vi "MUSIQC_trap_control.vi"() -> ()   [LabVIEW 2009]
uses:
  <vilib>/DAQmx/configure/timing.llb/DAQmx Timing (Implicit).vi
  <vilib>/DAQmx/create/channels.llb/DAQmx Create Channel (CO-Pulse Generation-Frequency).vi
  <vilib>/DAQmx/configure/timing.llb/DAQmx Timing (Sample Clock).vi
  <vilib>/DAQmx/create/channels.llb/DAQmx Create Channel (CI-Count Edges).vi
  <vilib>/DAQmx/read.llb/DAQmx Read (Counter U32 1Chan 1Samp).vi
  <vilib>/Utility/file.llb/Write To Spreadsheet File (I64).vi
  Program Files/National Instruments/LabVIEW 2009/resource/objmgr/daqmx.rc
  <vilib>/Analysis/NI_AALBase.lvlib
panel:
  out "Change with UV":i32(graph)
  in  "snap":bool
  in  "Threshold":u32
  in  "Auto Load":bool
  in  "Oven":bool
  in  "UV":bool=TRUE
  in  "UV Interval (s)":dbl
  in  "RF":bool
  in  "Blue":bool
  in  "Red":bool
  out "Mean/Variance":dbl
  out "Variance":dbl format="%0.2f"
  out "Mean":dbl format="%0.2f"
  in  "Samples per block":i32=100 min=1 step=1
  in  "Sample Time":dbl=0.02 step=0.0001
  in  "stop":bool
  out "PMT Counts":cluster{"mean":dbl, u32, i32}(graph)
  out "Counts total":dbl
  # "Trap 1"
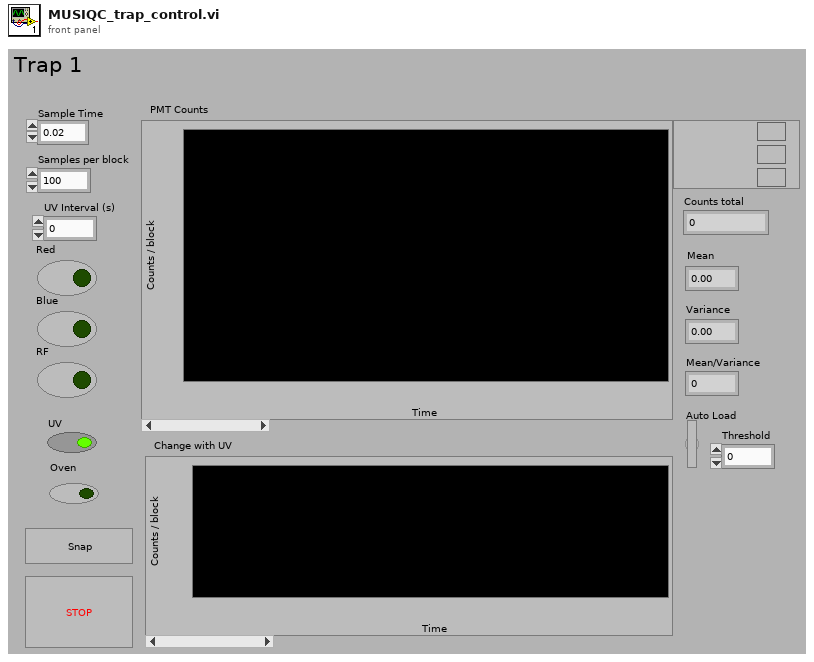
[diagram p1: front panel]
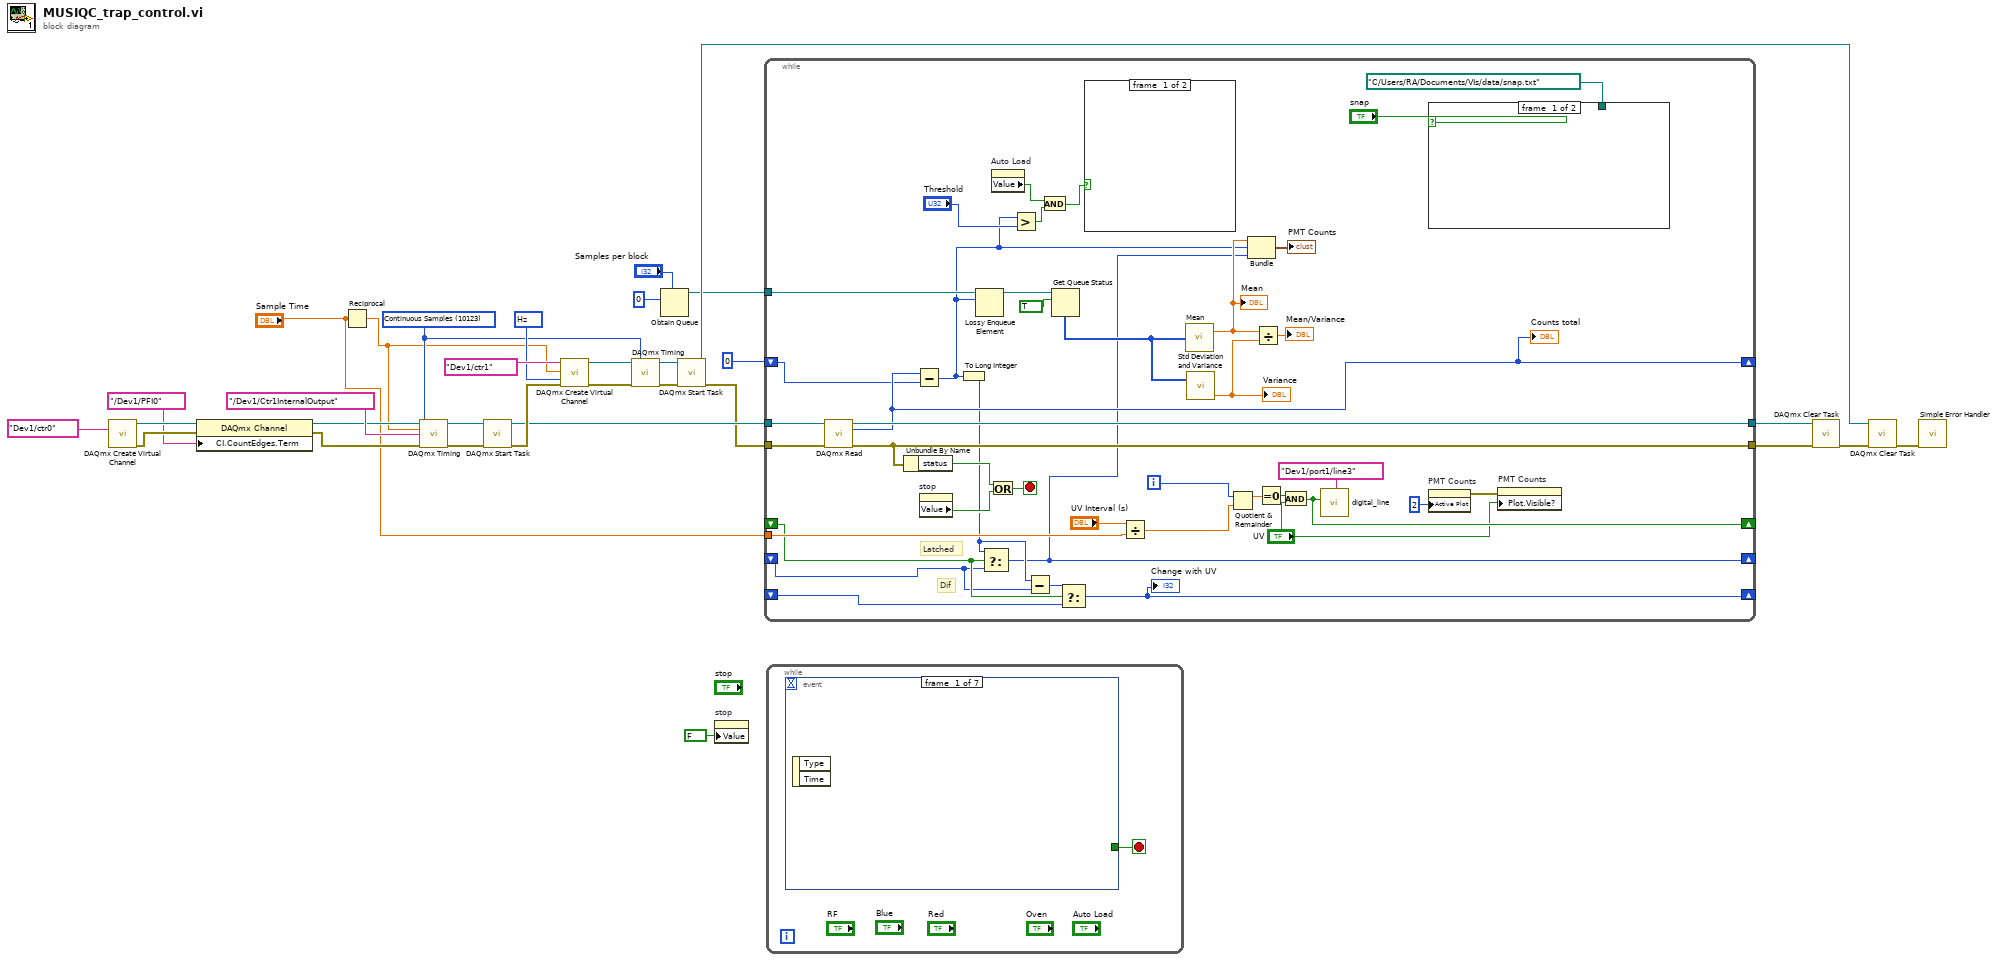
[diagram p0: block diagram]
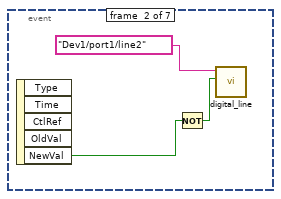
[diagram p2: hidden frame]
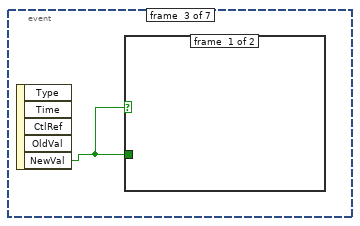
[diagram p3: hidden frame]
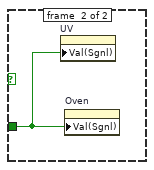
[diagram p4: hidden frame]
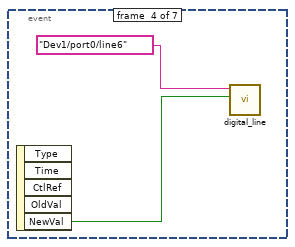
[diagram p5: hidden frame]
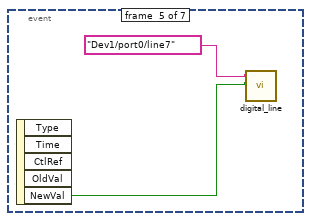
[diagram p6: hidden frame]
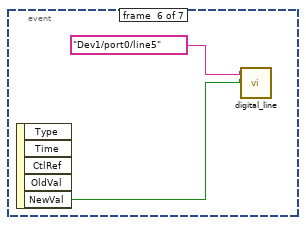
[diagram p7: hidden frame]
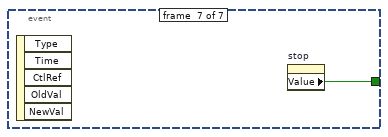
[diagram p8: hidden frame]
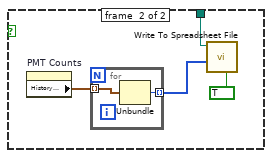
[diagram p9: hidden frame]
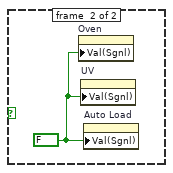
[diagram p10: hidden frame]
diagram:
  w27 = 10373 items=["Hz"=10373] ("units")
  w3 = 10123 items=["Finite Samples"=10178, "Continuous Samples"=10123, "Hardware Timed Single Point"=12522] ("sample mode")
  n1 = call-poly <vilib>:"DAQmx Create Virtual Channel.vi"("counter"=tag "Dev1/ctr0") -> ("task out"=w12:refnum<k21>, "error out"=w11:errorcluster)  [unwired: 13 in]
  n2 = property class="DAQmx Channel"(reference=w12, error in=w11, "CI.CountEdges.Term"=tag "/Dev1/PFI0") -> (reference out=w14:refnum<k21>, error out=w13:errorcluster)
  n3 = Reciprocal(x="Sample Time") -> (1/x=w2:dbl)
  n4 = call-poly <vilib>:"DAQmx Timing.vi"("task/channels in"=w14, "sample mode"=w3, "rate"=w2, "source"=tag "/Dev1/Ctr1InternalOutput", "error in"=w13) -> ("task out"=w30:refnum<k21>, "error out"=w29:errorcluster)  [unwired: 9 in]
  n5 = call <vilib>:"DAQmx Start Task.vi"("task/channels in"=w30, "error in"=w29) -> ("task out"=w17:refnum<k21>, "error out"=w21:errorcluster)  [unwired: 12 in]
  n6 = call-poly <vilib>:"DAQmx Create Virtual Channel.vi"("frequency"=w2, "counter"=tag "Dev1/ctr1", "units"=w27, "error in"=w21) -> ("task out"=w25:refnum<k21>, "error out"=w24:errorcluster)  [unwired: 10 in]
  n7 = call-poly <vilib>:"DAQmx Timing.vi"("task/channels in"=w25, "sample mode"=w3, "error in"=w24) -> ("task out"=w23:refnum<k21>, "error out"=w22:errorcluster)  [unwired: 11 in]
  n8 = Obtain Queue(max queue size (-1, unlimited)="Samples per block", element data type=u32 0) -> (queue out=w7:refnum<queue>)  [unwired: 3 in, 2 out]
  n9 = call <vilib>:"DAQmx Start Task.vi"("task/channels in"=w23, "error in"=w22) -> ("task out"=w16:refnum<k21>, "error out"=w15:errorcluster)  [unwired: 12 in]
  n10 = property on="stop" class="Bool (strict)"("Value"=FALSE ("stop")) -> ()  [unwired: 2 in, 2 out]
  n11 = while {
    shift-right: [w44] -> _
    shift-left: u32 0 -> [w43]
    tunnel: [w71] -> w19
    tunnel: [w70] -> w18
    tunnel: w17 -> [w69]
    tunnel: w15 -> [w68]
    tunnel: w7 -> [w67]
    tunnel: "Sample Time" -> [w48]
    shift-right: [w45] -> _
    shift-left: _ -> [w42]
    shift-right: [w34] -> _
    shift-left: _ -> [w41]
    shift-right: [w39] -> _
    shift-left: _ -> [w37]
    i -> [w49]
    stop <- w73 stop-if-true
    # "Dif"
    # "Latched"
    n12 = call-poly <vilib>:"DAQmx Read.vi"("task/channels in"=w69, "error in"=w68) -> ("task out"=w70:refnum<k21>, "data"=w44:u32, "error out"=w71:errorcluster)  [unwired: 11 in]
    "Counts total" <- w44
    n13 = Unbundle By Name(w71) -> ("status"=w72:bool)
    n14 = Subtract(x=w44, y=w43) -> (x-y=w35:u32)
    n15 = property on="stop" class="Bool (strict)"() -> ("Value"=w60:bool)  [unwired: 2 in, 2 out]
    n16 = To Long Integer(number=w35) -> (32bit integer=w38:i32)
    n17 = Lossy Enqueue Element(queue=w67, element=w35) -> (queue out=w66:refnum<queue>)  [unwired: 1 in, 3 out]
    n18 = Select(t=w38, s=w42, f=w41) -> (s? t:f=w34:i32)
    n19 = Or(x=w72, y=w60) -> (x .or. y?=w73:bool)
    n20 = property on="Auto Load" class="Bool (strict)"() -> ("Value"=w57:bool)  [unwired: 2 in, 2 out]
    n21 = Greater?(x=w35, y="Threshold") -> (0:w58:bool)
    n22 = Subtract(x=w38, y=w41) -> (x-y=w40:i32)
    n23 = And(x=w57, y=w58) -> (x .and. y?=w56:bool)
    n24 = Get Queue Status(queue=w66, return elements? (F)=TRUE) -> (elements=w54:u32[])  [unwired: 1 in, 7 out]
    n25 = Select(t=w40, s=w42, f=w37) -> (s? t:f=w39:i32)
    "Change with UV" <- w39
    n26 = case shown="True" w56 {
      frame #0 {
      }
      frame #1 {
        w80 = FALSE ("Auto Load")
        n27 = property on="Oven" class="Bool (strict)"("Val(Sgnl)"=w80) -> ()  [unwired: 2 in, 2 out]
        n28 = property on="UV" class="Bool (strict)"("Val(Sgnl)"=w80) -> ()  [unwired: 2 in, 2 out]
        n29 = property on="Auto Load" class="Bool (strict)"("Val(Sgnl)"=w80) -> ()  [unwired: 2 in, 2 out]
      }
    }
    n30 = Divide(x="UV Interval (s)", y=w48) -> (x/y=w47:dbl)
    n31 = call <vilib>:"Mean.vi"("X"=w54) -> ("mean"=w61:dbl)  [unwired: 1 out]
    "Mean" <- w61
    n32 = call <vilib>:"Std Deviation and Variance.vi"("X"=w54) -> ("variance"=w64:dbl)  [unwired: 1 in, 2 out]
    "Variance" <- w64
    n33 = Quotient & Remainder(x=w49, y=w47) -> (x-y*floor(x/y)=w52:dbl)  [unwired: 1 out]
    n34 = Bundle("mean"=w61, w35, w34) -> (→"PMT Counts":cluster{"mean":dbl, u32, i32})  [unwired: 1 in]
    n35 = Divide(x=w61, y=w64) -> (x/y=→"Mean/Variance":dbl)
    n36 = Equal To 0?(x=w52) -> (x = 0?=w50:bool)
    n37 = And(x=w50, y="UV") -> (x .and. y?=w45:bool)
    n38 = call "digital_line.vi"("NewVal"=w45, "lines"=tag "Dev1/port1/line3") -> ()  [unwired: 2 in]
    n39 = property on="PMT Counts" class="WFChart (strict)"("Active Plot"=u32 2) -> (error out=w32:errorcluster)  [unwired: 2 in, 1 out]
    n40 = case shown="True" "snap" {
      tunnel: path "C:/Users/RA/Documents/VIs/data/snap.txt" ("file path (dialog if empty)") -> [_ w76]
      frame #0 {
      }
      frame #1 {
        n41 = property on="PMT Counts" class="WFChart (strict)"() -> ("History Data"=w75:cluster{"mean":dbl, u32, i32}[])  [unwired: 2 in, 2 out]
        n42 = for {
          tunnel: w75 -> [w79] mode=indexing
          tunnel: [w78] -> w74 mode=indexing
          n43 = Unbundle(w79) -> (w78:u32)  [unwired: 2 out]
        }
        n44 = call-poly <vilib>:"Write To Spreadsheet File.vi"("transpose? (no:F)"=TRUE, "1D data"=w74, "file path (dialog if empty)"=w76) -> ()  [unwired: 5 in, 1 out]
      }
    }
    n45 = property on="PMT Counts" class="WFChart (strict)"(error in=w32, "Plot.Visible?"="UV") -> ()  [unwired: 1 in, 2 out]
  }
  n46 = while {
    stop <- w81 stop-if-true
    n47 = event shown="[3] \"Red\": Value Change" {
      selector: _ -> [_ _ _ _ _ _ _]
      dyn-events: _ -> [_ _ _ _ _ _ _]
      timeout: _ -> [_ _ _ _ _ _ _]
      tunnel: [_ _ _ _ _ _ w93] -> w81
      event #0 {
        n48 = event-data() -> ()  [unwired: 1 in, 2 out]
      }
      event #1 {
        n49 = event-data() -> ("NewVal"=w83:bool)  [unwired: 1 in, 4 out]
        n50 = Not(x=w83) -> (.not. x?=w82:bool)
        n51 = call "digital_line.vi"("NewVal"=w82, "lines"=tag "Dev1/port1/line2") -> ()  [unwired: 2 in]
      }
      event #2 {
        n52 = event-data() -> ("NewVal"=w85:bool)  [unwired: 1 in, 4 out]
        n53 = case shown="True" w85 {
          tunnel: w85 -> [_ w86]
          frame #0 {
          }
          frame #1 {
            n54 = property on="UV" class="Bool (strict)"("Val(Sgnl)"=w86) -> ()  [unwired: 2 in, 2 out]
            n55 = property on="Oven" class="Bool (strict)"("Val(Sgnl)"=w86) -> ()  [unwired: 2 in, 2 out]
          }
        }
      }
      event #3 {
        n56 = event-data() -> ("NewVal"=w87:bool)  [unwired: 1 in, 4 out]
        n57 = call "digital_line.vi"("NewVal"=w87, "lines"=tag "Dev1/port0/line6") -> ()  [unwired: 2 in]
      }
      event #4 {
        n58 = event-data() -> ("NewVal"=w89:bool)  [unwired: 1 in, 4 out]
        n59 = call "digital_line.vi"("NewVal"=w89, "lines"=tag "Dev1/port0/line7") -> ()  [unwired: 2 in]
      }
      event #5 {
        n60 = event-data() -> ("NewVal"=w91:bool)  [unwired: 1 in, 4 out]
        n61 = call "digital_line.vi"("NewVal"=w91, "lines"=tag "Dev1/port0/line5") -> ()  [unwired: 2 in]
      }
      event #6 {
        n62 = event-data() -> ()  [unwired: 1 in, 5 out]
        n63 = property on="stop" class="Bool (strict)"() -> ("Value"=w93:bool)  [unwired: 2 in, 2 out]
      }
    }
  }
  n64 = call <vilib>:"DAQmx Clear Task.vi"("task in"=w18, "error in"=w19) -> ("error out"=w6:errorcluster)  [unwired: 13 in]
  n65 = call <vilib>:"DAQmx Clear Task.vi"("task in"=w16, "error in"=w6) -> ("error out"=w5:errorcluster)  [unwired: 13 in]
  n66 = call <vilib>:"Simple Error Handler.vi"("error in (no error)"=w5) -> ()  [unwired: 4 in, 5 out]
